vi "Scope.vi"(0 "Array":waveform(i16)[](array[waveform])) -> ()   [LabVIEW 2010]
uses:
  70user.lib/TheSigTab.vi
panel:
  in  "SigList":cluster{bool, string}[](array[cluster]) caption="Каналы АЦП"
  out "Waveform Graph":waveform(i16)[](graph)
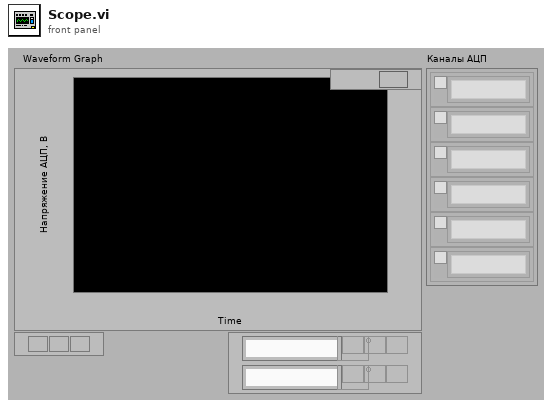
[diagram p1: front panel]
types:
  T1 = cluster{"s_Type":u16, "FIFO":u16, "IrqStep":u16, "Pages":u16, "AutoInit":u16, "dRate":dbl, "dKadr":dbl, "dScale":dbl, "Rate":u16, "Kadr":u16, "Scale":u16, "FPDelay":u16, "SynchroType":u16, "SynchroSensitivity":u16, "SynchroMode":u16, "AdChannel":u16, "AdPorog":u16, "NCh":u16, "Chn":i32[], "IrqEna":u16, "AdcEna":u16}
  T2 = cluster{"Сигнал":string, "Тип":enum16{"Напряжение/Ток", "ЧР", "Температура", "Давление"}, "Object":string}[]
  T3 = cluster{"Сигнал":string, "Тип":enum16{"Напряжение/Ток", "ЧР", "Температура", "Давление"}, "Object":string}
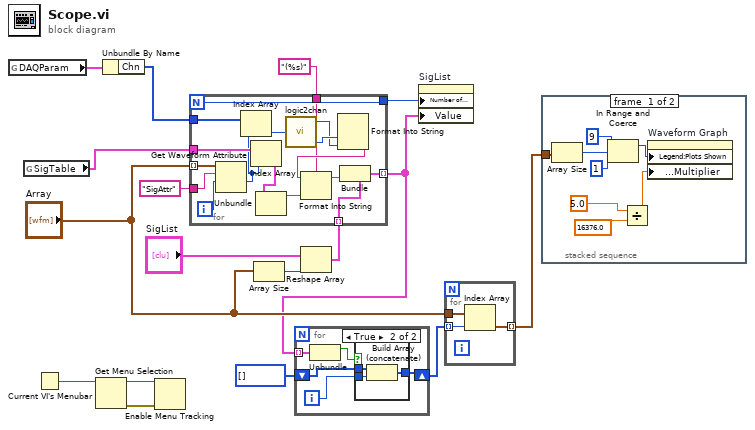
[diagram p0: block diagram]
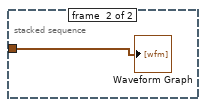
[diagram p2: hidden frame]
diagram:
  n1 = global read "TheSigTab.vi" "DAQParam"() -> (w6:T1)
  n2 = global read "TheSigTab.vi" "SigTable"() -> (w11:T2)
  n3 = Current VI's Menubar() -> (w10:refnum<k9>)
  n4 = Get Menu Selection(0:w10) -> (5:w9:refnum<k9>, 8:w8:errorcluster)  [unwired: 3 in, 3 out]
  n5 = Unbundle By Name(w6) -> ("Chn"=w5:i32[])
  n6 = Enable Menu Tracking(2:w8, 4:w9) -> ()  [unwired: 1 in, 2 out]
  n7 = Array Size(array="Array") -> (size(s)=w13:i32)
  n8 = Reshape Array("SigList", w13) -> (w14:cluster{bool, string}[])
  n9 = for {
    N -> [w31]
    tunnel: "Array" -> [w34] mode=indexing
    tunnel: "SigAttr" -> [w33]
    tunnel: [w32] -> w3 mode=indexing
    tunnel: [w31] -> w16
    tunnel: w14 -> [w30] mode=indexing
    tunnel: w11 -> [w28]
    tunnel: w5 -> [w26]
    tunnel: "(%s)" -> [w18]
    i -> [w29]
    n10 = Get Waveform Attribute(5:w29, 6:w33, 7:w34) -> (1:w25:i32)  [unwired: 1 in, 3 out]
    n11 = Index Array(array=w26, index=w25) -> (element=w24:i32)
    n12 = Index Array(array=w28, index=w25) -> (element=w27:T3)
    n13 = Unbundle(w27) -> ("Сигнал"=w21:string)  [unwired: 2 out]
    n14 = call "logic2chan.vi"("value"=w24) -> ("Канал"=w22:u8, "Switch"=w23:enum16{"X-Y", "На землю", "X", "Y"})  [unwired: 1 out]
    n15 = Format Into String(w23, w22) -> (resulting string=w19:string)  [unwired: 3 in, 1 out]
    n16 = Format Into String(format string=w18, initial string=w19, w21) -> (resulting string=w20:string)  [unwired: 1 in, 1 out]
    n17 = Bundle(cluster=w30, w20) -> (w32:cluster{bool, string})  [unwired: 1 in]
  }
  n18 = for {
    tunnel: w3 -> [w39] mode=indexing
    shift-right: [w36] -> w4
    shift-left: i32[] [] -> [w35]
    i -> [w37]
    n19 = Unbundle(w39) -> (w38:bool)  [unwired: 1 out]
    n20 = case shown="True" w38 {
      tunnel: w37 -> [_ w43]
      tunnel: [w40 w42] -> w36
      tunnel: w35 -> [w40 w41]
      frame False {
      }
      frame True {
        n21 = Build Array (concatenate)(w41, w43) -> (w42:i32[])
      }
    }
  }
  n22 = property on="SigList" class="Arr (strict)"("Number of Rows"=w16, "Value"=w3) -> ()  [unwired: 2 in, 2 out]
  n23 = for {
    tunnel: "Array" -> [w46]
    tunnel: [w44] -> w1 mode=indexing
    tunnel: w4 -> [w45] mode=indexing
    n24 = Index Array(array=w46, index=w45) -> (element=w44:waveform(i16))
  }
  n25 = stacked-sequence {
    tunnel: w1 -> [w51 w55]
    frame #0 {
      n26 = Array Size(array=w51) -> (size(s)=w52:i32)
      n27 = In Range and Coerce(upper limit=9, x=w52, lower limit=1) -> (coerced(x)=w50:i32)  [unwired: 1 out]
      n28 = Divide(x=5.0, y=16376.0) -> (x/y=w47:dbl)
      n29 = property on="Waveform Graph" class="WFGraph (strict)"("Legend:Plots Shown"=w50, "Y Scale.Offset and Multiplier:Multiplier"=w47) -> ()  [unwired: 2 in, 2 out]
    }
    frame #1 {
      "Waveform Graph" <- w55
    }
  }
